vi "Python@File__Parameter.vi"(1 "ParamterIn":string) -> (0 "ParamterOut":string)   [LabVIEW 2019]
uses:
  MainFrame/Global.vi
panel:
  in  "FileName":string(combo)
  in  "Confirm":bool
  # "Python@File $PythonFile"
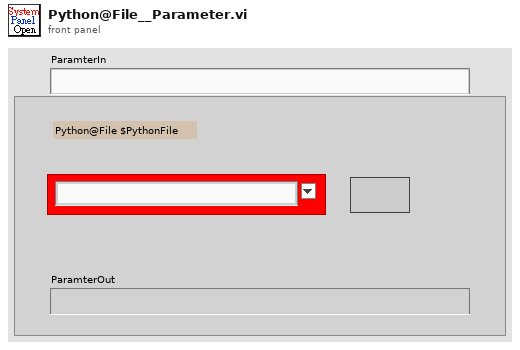
[diagram p1: front panel]
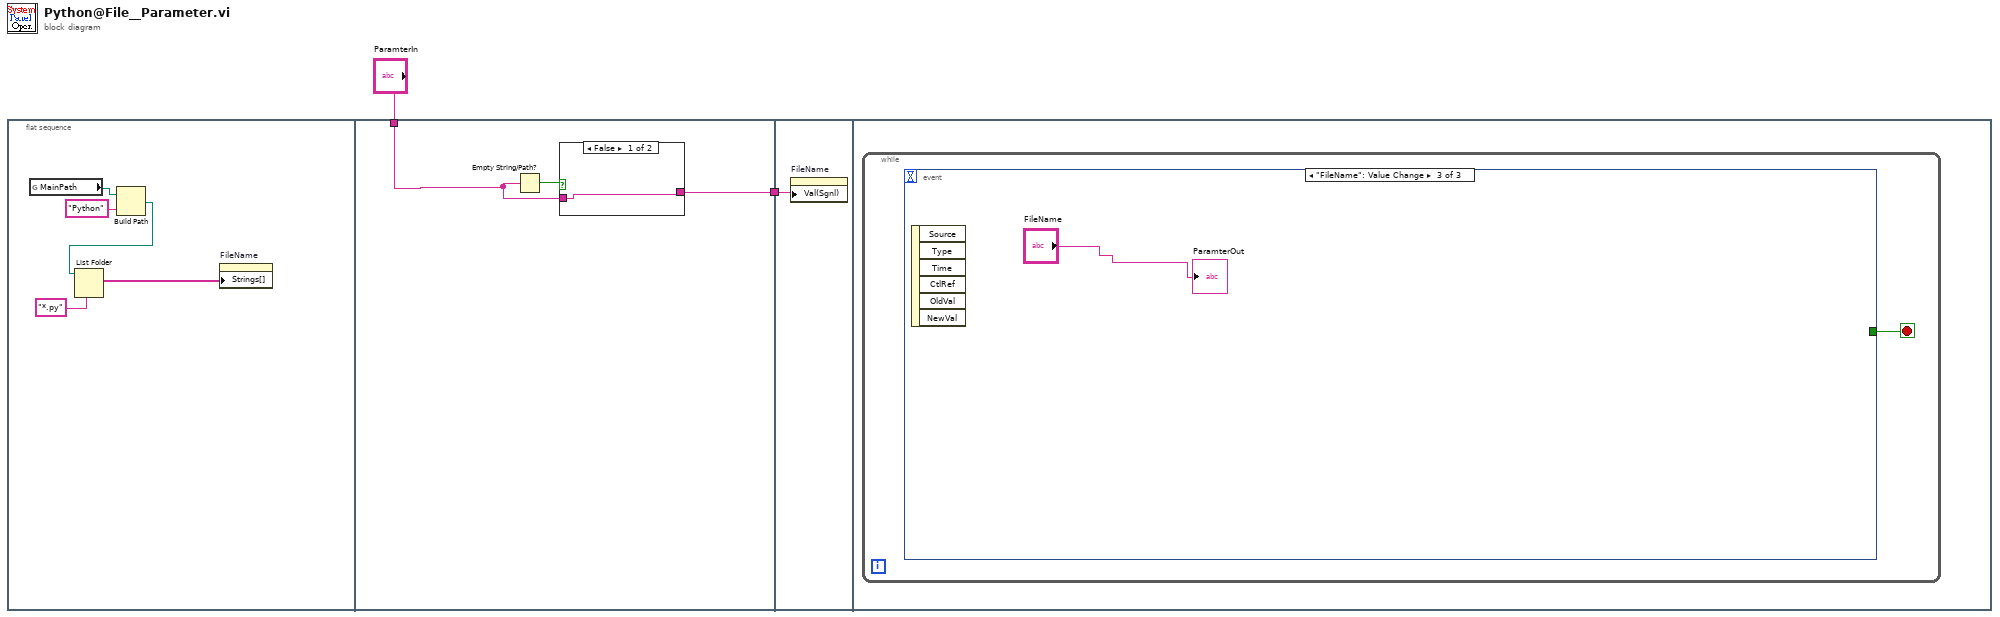
[diagram p0: block diagram]
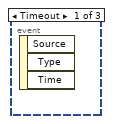
[diagram p3: hidden frame]
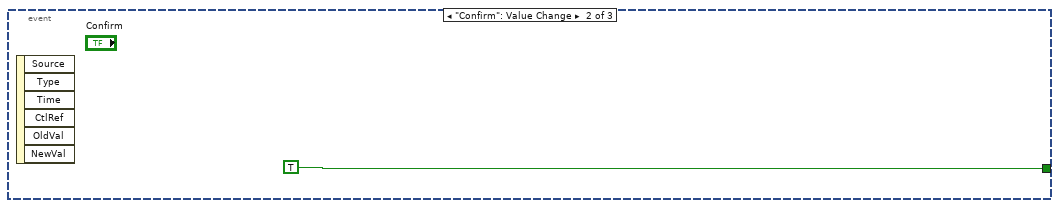
[diagram p4: hidden frame]
diagram:
  n1 = flat-sequence {
    tunnel: "ParamterIn" -> [w8]
    tunnel: [w9] -> w1
    tunnel: w1 -> [w13]
    frame #0 {
      n2 = global read "Global.vi" "MainPath"() -> (w5:path)
      n3 = Build Path(base path=w5, name or relative path="Python") -> (appended path=w3:path)
      n4 = List Folder(path=w3, pattern="*.py") -> (filenames=w6:string[])  [unwired: 2 in, 3 out]
      n5 = property on="FileName" class="CmbBox"("Strings[]"=w6) -> ()  [unwired: 2 in, 2 out]
    }
    frame #1 {
      n6 = Empty String/Path?(string/path=w8) -> (empty?=w10:bool)
      n7 = case shown="False" w10 {
        tunnel: w8 -> [w11 w12]
        tunnel: [w11 w12] -> w9
        frame False {
        }
        frame True {
        }
      }
    }
    frame #2 {
      n8 = property on="FileName" class="CmbBox"("Val(Sgnl)"=w13) -> ()  [unwired: 2 in, 2 out]
    }
    frame #3 {
      n9 = while {
        stop <- w14 stop-if-true
        n10 = event shown="[2] \"FileName\": Value Change" {
          selector: _ -> [_ _ _]
          dyn-events: _ -> [_ _ _]
          timeout: _ -> [_ _ _]
          tunnel: [_ TRUE _] -> w14
          event Timeout {
            n11 = event-data() -> ()  [unwired: 1 in, 3 out]
          }
          event "Confirm": Value Change {
            n12 = event-data() -> ()  [unwired: 1 in, 6 out]
          }
          event "FileName": Value Change {
            n13 = event-data() -> ()  [unwired: 1 in, 6 out]
            "ParamterOut" <- "FileName"
          }
        }
      }
    }
  }
